vi "Stop Core.vi"(10 "final error code":i32, 11 "Server Controller in":refnum<class "Server Controller.lvclass">) -> (3 "Server Controller out":refnum<class "Server Controller.lvclass">)   [LabVIEW 2026, in "Server Controller.lvlib" / "Server Controller.lvclass"]
uses:
  Server Controller.lvclass
  Server Controller.lvclass/Server Controller.ctl
  <vilib>/ActorFramework/Message Enqueuer/Message Enqueuer.lvclass/Message Enqueuer.ctl
  <vilib>/ActorFramework/Message Enqueuer/Enqueue.vi
  <vilib>/ActorFramework/Stop Msg/Stop Msg.lvclass
  C:/Program Files/National Instruments/LabVIEW 2026/vi.lib/ActorFramework/Message/Message.lvclass
  <vilib>/ActorFramework/Message Priority Queue/Priority Enqueue.vi
  framework/Controller/Controller.lvclass
  <vilib>/ActorFramework/Message Enqueuer/Message Enqueuer.lvclass
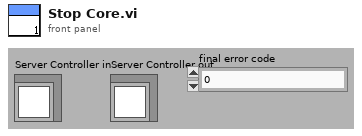
[diagram p1: front panel]
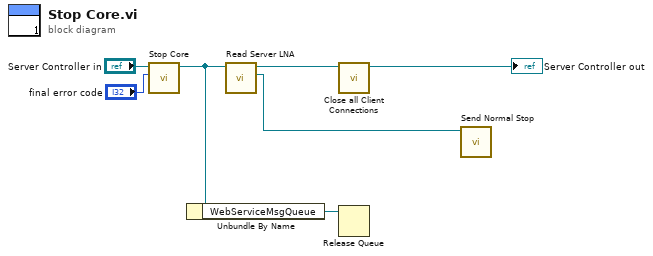
[diagram p0: block diagram]
diagram:
  n1 = call-parent "Stop Core.vi"("final error code"="final error code", "Controller in"="Server Controller in") -> ("Controller out"=w2:refnum<class "Server Controller.lvclass">)  [unwired: 9 in]
  n2 = Unbundle By Name(w2) -> ("WebServiceMsgQueue"=w1:refnum<queue>)
  n3 = call "Read Server LNA.vi"("Server Controller in"=w2) -> ("Actor Framework:Message Enqueuer"=w3:refnum<class "Message Enqueuer.lvclass">, "Server Controller out"=w5:refnum<class "Server Controller.lvclass">)  [unwired: 8 in, 1 out]
  n4 = call "Close all Client Connections.vi"("Server Controller in"=w5) -> ("Server Controller out"=→"Server Controller out":refnum<class "Server Controller.lvclass">)  [unwired: 10 in]
  n5 = Release Queue(queue=w1) -> ()  [unwired: 2 in, 3 out]
  n6 = call <vilib>:"Send Normal Stop.vi"("Message Enqueuer"=w3) -> ()  [unwired: 10 in, 1 out]
